vi "Test Sound.vi"() -> ()   [LabVIEW 2021, in "Sounds.lvlib"]
uses:
  Sounds.lvlib
  Sounds/Sounds.lvclass
  C:/Program Files/National Instruments/LabVIEW 2024/vi.lib/ActorFramework/Actor/Actor.lvclass
  Sounds/Sounds.lvclass/Sounds.ctl
  <vilib>/ActorFramework/Actor/Actor.lvclass
panel:
  in  "Sound File Path":path=path "C:/Users/ekerry/Documents/challenge-of-champions/Sounds/Clips/jeopardy-board-sms.wav"
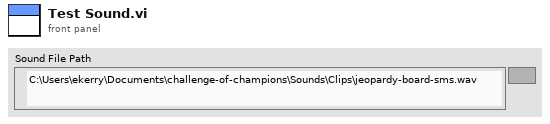
[diagram p1: front panel]
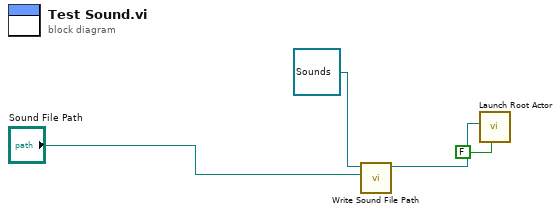
[diagram p0: block diagram]
diagram:
  n1 = call "Write Sound File Path.vi"("Sound File Path"="Sound File Path", "Sounds in"=refnum<class "Sounds.lvclass"> refnum ("Sounds.lvlib:Sounds.lvclass")) -> ("Sounds out"=w3:refnum<class "Sounds.lvclass">)  [unwired: 8 in, 1 out]
  n2 = call <vilib>:"Launch Root Actor.vi"("Open Actor Core front panel? (F)"=FALSE, "Actor"=w3) -> ()  [unwired: 8 in, 2 out]
